vi "Has Gear.vi"(8 "error in":errorcluster) -> (0 "error out":errorcluster, 3 "Has Gear?":bool)   [LabVIEW 2016, in "Intake.lvlib"]
uses:
  Intake.lvlib
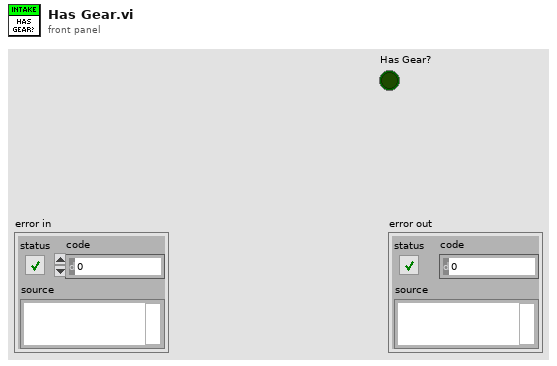
[diagram p1: front panel]
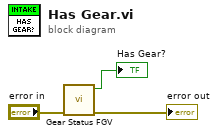
[diagram p0: block diagram]
diagram:
  n1 = call "Gear Status FGV.vi"("error in (no error)"="error in") -> ("error out"=→"error out":errorcluster, "Has Gear?"=→"Has Gear?":bool)  [unwired: 8 in, 1 out]
